vi "Kai.vi"(11 "Vision Results":T1={"Distance (ft)"=15.49734580202351, "Score"=91.78787878787878, "Normalized"={"Center"={0.14657821229050283, -0.025232774674115444}, "Rectangle"={"Numeric"=0.07499999999999996, "Numeric 2"=0.008333333333333304, "Numeric 3"=0.2250000000000001, "Numeric 5"=-0.17500000000000004}}, "Pixels"={"Center"={183.45251396648044, 123.02793296089385}, "Rectangle"={"Numeric"=172.0, "Numeric 2"=119.0, "Numeric 3"=196.0, "Numeric 5"=141.0}}}) -> ()   [LabVIEW 2016]
uses:
  Robot Global Data.vi
  <vilib>/Rock Robotics/Network Tables/NT Write Boolean.vi
panel:
  in  "lower limit":dbl=-110.0 format="%#_13g"
  in  "upper limit":dbl=110.0 format="%#_13g"
  in  "b-value (RPM)":dbl=1475.0
  in  "X-value (RPM)":dbl=250.0
  out "RPM":dbl=5349.336450505878
  out "Distance (ft)":dbl=15.49734580202351
  in  "Camera center (px)":dbl=183.0 format="%#_13g"
  in  "Dg per px":dbl=0.45 format="%#_13g"
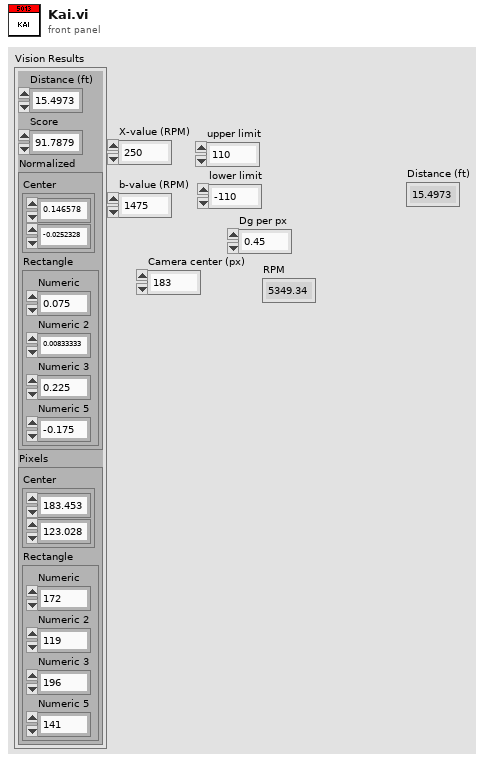
[diagram p1: front panel]
types:
  T1 = cluster{"Distance (ft)":dbl, "Score":dbl, "Normalized":cluster{"Center":cluster{dbl, dbl}, "Rectangle":cluster{"Numeric":dbl, "Numeric 2":dbl, "Numeric 3":dbl, "Numeric 5":dbl}}, "Pixels":cluster{"Center":cluster{dbl, dbl}, "Rectangle":cluster{"Numeric":dbl, "Numeric 2":dbl, "Numeric 3":dbl, "Numeric 5":dbl}}}
  T2 = cluster{"Center":cluster{dbl, dbl}, "Rectangle":cluster{"Numeric":dbl, "Numeric 2":dbl, "Numeric 3":dbl, "Numeric 5":dbl}}
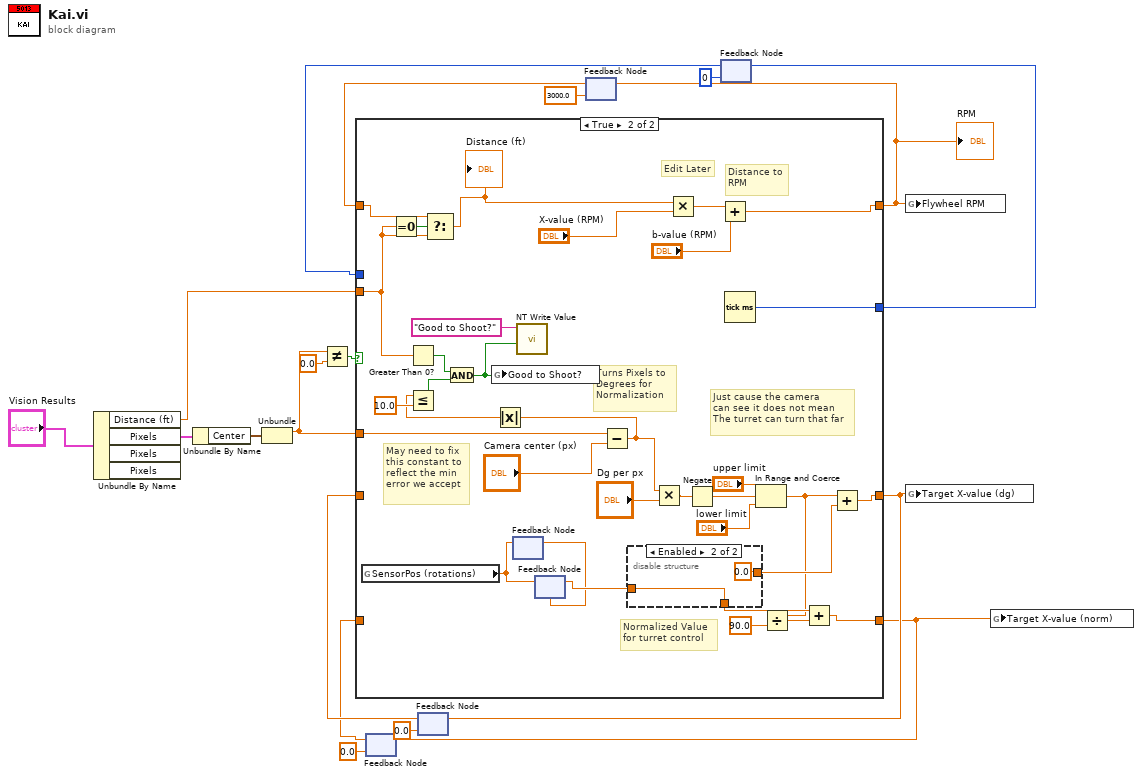
[diagram p0: block diagram]
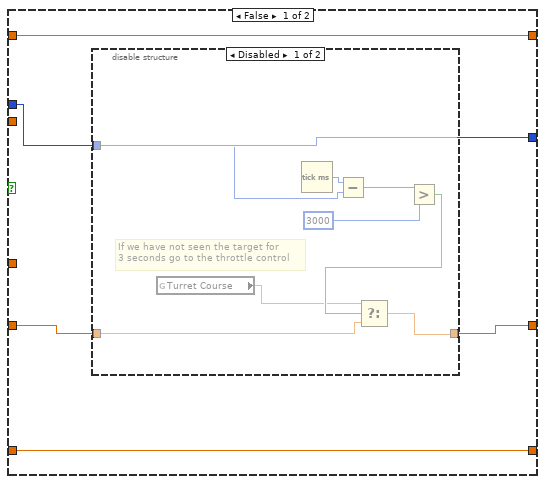
[diagram p2: hidden frame]
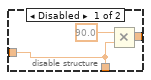
[diagram p4: hidden frame]
diagram:
  n1 = Unbundle By Name("Vision Results") -> ("Distance (ft)"=w1:dbl, "Pixels"=w19:T2)  [unwired: 2 out]
  n2 = Unbundle By Name(w19) -> ("Center"=w18:cluster{dbl, dbl})
  n3 = Unbundle(w18) -> (w14:dbl)  [unwired: 1 out]
  n4 = Not Equal?(x=w14, y=0.0) -> (x != y?=w16:bool)
  n5 = feedback #1(0.0) -> (w9:dbl)
  n6 = feedback #2(0.0) -> (w15:dbl)
  n7 = feedback #3(3000.0) -> (w13:dbl)
  n8 = feedback #4(u32 0 ("millisecond timer value")) -> (w4:u32)
  n9 = case shown="True" w16 {
    tunnel: w15 -> [w21 _]
    tunnel: w14 -> [_ w48]
    tunnel: [w20 w60] -> w12
    tunnel: w1 -> [_ w40]
    tunnel: [w23 w34] -> w2
    tunnel: w13 -> [w23 w42]
    tunnel: [w24 w57] -> w10
    tunnel: w9 -> [w24 _]
    tunnel: w4 -> [w22 _]
    tunnel: [w22 w49] -> w5
    frame False {
      n10 = disable-structure shown="Disabled" {
        disable-tunnel: w22 -> [w31 _]
        disable-tunnel: w21 -> [w28 w33]
        disable-tunnel: [w27 w33] -> w20
        frame Disabled {
          # "If we have not seen the target for \n3 seconds go to the throttle control"
          n11 = global read "Robot Global Data.vi" "Turret Course"() -> (w25:dbl)
          n12 = Tick Count (ms)() -> (millisecond timer value=w32:u32)
          n13 = Subtract(x=w32, y=w31) -> (x-y=w30:u32)
          n14 = Greater?(x=w30, y=u32 3000) -> (0:w26:bool)
          n15 = Select(t=w25, s=w26, f=w28) -> (s? t:f=w27:dbl)
        }
        frame Enabled {
        }
      }
    }
    frame True {
      # "May need to fix\nthis constant to\nreflect the min \nerror we accept"
      # "Just cause the camera \ncan see it does not mean\nThe turret can turn that far"
      # "Normalized Value\nfor turret control"
      # "Edit Later"
      # "Turns Pixels to \nDegrees for \nNormalization"
      # "Distance to\nRPM"
      n16 = global read "Robot Global Data.vi" "SensorPos (rotations)"() -> (w55:dbl)
      n17 = Equal To 0?(x=w40) -> (x = 0?=w41:bool)
      n18 = Greater Than 0?(x=w40) -> (x > 0?=w45:bool)
      n19 = Select(t=w42, s=w41, f=w40) -> (s? t:f=w37:dbl)
      "Distance (ft)" <- w37
      n20 = feedback-in #5(w55) -> ()
      n21 = feedback #5() -> (w53:dbl)  [unwired: 1 in]
      n22 = feedback #6(w53) -> (w54:dbl)
      n23 = feedback-in #6(w55) -> ()
      n24 = Subtract(x=w48, y="Camera center (px)") -> (x-y=w44:dbl)
      n25 = Absolute Value(x=w44) -> (abs(x)=w43:dbl)
      n26 = Less Or Equal?(x=w43, y=10.0) -> (x <= y?=w46:bool)
      n27 = And(x=w45, y=w46) -> (x .and. y?=w38:bool)
      n28 = global write "Robot Global Data.vi" "Good to Shoot?"(w38) -> ()
      n29 = call-poly <vilib>:"NT Write Value.vi"("Boolean"=w38, "Name"="Good to Shoot?") -> ()  [unwired: 9 in, 1 out]
      n30 = disable-structure shown="Enabled" {
        disable-tunnel: [w67 w71] -> w61
        disable-tunnel: [w68 0.0] -> w59
        disable-tunnel: w54 -> [w67 w71]
        frame Disabled {
          n31 = Multiply(x=90.0, y=w67) -> (x*y=w68:dbl)
        }
        frame Enabled {
        }
      }
      n32 = Multiply(x=w44, y="Dg per px") -> (x*y=w58:dbl)
      n33 = Multiply(x=w37, y="X-value (RPM)") -> (x*y=w64:dbl)
      n34 = Negate(x=w58) -> (-x=w56:dbl)
      n35 = Add(x=w64, y="b-value (RPM)") -> (x+y=w34:dbl)
      n36 = Tick Count (ms)() -> (millisecond timer value=w49:u32)
      n37 = In Range and Coerce(upper limit="upper limit", x=w56, lower limit="lower limit") -> (coerced(x)=w52:dbl)  [unwired: 1 out]
      n38 = Divide(x=w52, y=90.0) -> (x/y=w62:dbl)
      n39 = Add(x=w61, y=w62) -> (x+y=w57:dbl)
      n40 = Add(x=w52, y=w59) -> (x+y=w60:dbl)
    }
  }
  "RPM" <- w2
  n41 = feedback-in #1(w10) -> ()
  n42 = feedback-in #2(w12) -> ()
  n43 = feedback-in #3(w2) -> ()
  n44 = feedback-in #4(w5) -> ()
  n45 = global write "Robot Global Data.vi" "Flywheel RPM"(w2) -> ()
  n46 = global write "Robot Global Data.vi" "Target X-value (dg)"(w12) -> ()
  n47 = global write "Robot Global Data.vi" "Target X-value (norm)"(w10) -> ()
